vi "MainV1.vi"() -> ()   [LabVIEW 2016]
uses:
  Control/GUICluster.ctl
  Control/Fahrart.ctl
  <vilib>/myRIO/Instrument Drivers/Onboard IO/AI/typedefs/AI Reference.ctl
  <vilib>/myRIO/Common/Instrument Driver Framework/Utilities/typedefs/myRIO Generic Hardware Reference.ctl
  <vilib>/myRIO/Common/Instrument Driver Framework/Utilities/typedefs/Hardware Version Enum.ctl
  <vilib>/myRIO/Common/Instrument Driver Framework/Utilities/typedefs/myRIO v1.0 Reference.ctl
  <vilib>/myRIO/Common/Instrument Driver Framework/Utilities/typedefs/Generic FPGA Reference.ctl
  <vilib>/myRIO/Common/Instrument Driver Framework/myRIO v1.0/AI/typedefs/AI Channels List.ctl
  <vilib>/myRIO/Common/Instrument Driver Framework/myRIO v1.0/AI/typedefs/AI Channels Enum.ctl
  <vilib>/myRIO/Common/Instrument Driver Framework/Utilities/typedefs/Analog Scaling Constants List.ctl
  <vilib>/myRIO/Common/Instrument Driver Framework/Utilities/typedefs/Analog Scaling Constants.ctl
  <vilib>/userdefined/High Color/nirio_resource_hc.ctl
  <vilib>/myRIO/Instrument Drivers/Onboard IO/PWM/typedefs/PWM Reference.ctl
  <vilib>/myRIO/Common/Instrument Driver Framework/myRIO v1.0/PWM/typedefs/PWM Channels Enum.ctl
  <vilib>/myRIO/Instrument Drivers/Onboard IO/PWM/typedefs/PWM Configuration.ctl
  <vilib>/myRIO/Common/Instrument Driver Framework/Utilities/vis/Is FPGA Ref Available.vi
  <vilib>/myRIO/Common/Instrument Driver Framework/myRIO v1.0/AI/vis/myRIO v1.1 Open AI.vi
  <vilib>/myRIO/Instrument Drivers/Onboard IO/AI/vis/Read.vi
  <vilib>/myRIO/Common/Instrument Driver Framework/myRIO v1.0/PWM/vis/myRIO v1.1 Open PWM.vi
  <vilib>/myRIO/Instrument Drivers/Onboard IO/PWM/vis/Set Duty Cycle and Frequency.vi
  <vilib>/myRIO/Common/Instrument Driver Framework/Utilities/vis/Validate Channels.vi
  <vilib>/myRIO/Common/Instrument Driver Framework/myRIO v1.0/AI/vis/myRIO v1.0 Reserve AI.vi
  <vilib>/myRIO/Common/Instrument Driver Framework/myRIO v1.0/PWM/vis/myRIO v1.0 Reserve PWM.vi
  <vilib>/myRIO/Common/Instrument Driver Framework/myRIO v1.0/AI/vis/myRIO v1.0 Build MUX Configuration AI.vi
  <vilib>/myRIO/Common/Instrument Driver Framework/myRIO v1.0/Resource Manager/vis/myRIO v1.0 Reserve Channel List.vi
  <vilib>/myRIO/Common/Instrument Driver Framework/myRIO v1.0/PWM/vis/myRIO v1.0 Build MUX Configuration PWM.vi
  <vilib>/myRIO/Common/Instrument Driver Framework/myRIO v1.0/Resource Manager/vis/myRIO v1.0 Reserve Channel.vi
  <vilib>/myRIO/Common/Instrument Driver Framework/myRIO v1.0/Resource Manager/vis/myRIO v1.0 Unreserve Channel.vi
  <vilib>/myRIO/Common/Instrument Driver Framework/myRIO v1.0/Resource Manager/vis/myRIO v1.0 Create Configuration List.vi
  <vilib>/myRIO/Common/Instrument Driver Framework/myRIO v1.0/Resource Manager/vis/myRIO v1.0 Build Mutex Name.vi
  <vilib>/Utility/VariantDataType/GetNumericInfo.vi
  <vilib>/Utility/error.llb/Error Cluster From Error Code.vi
  <vilib>/myRIO/Common/Instrument Driver Framework/myRIO v1.0/myRIO v1.1 Open.vi
  <vilib>/myRIO/Common/Instrument Driver Framework/Utilities/vis/IO Manager.vi
  <vilib>/myRIO/Common/Instrument Driver Framework/Utilities/vis/Configuration Manager.vi
  <vilib>/myRIO/Common/Instrument Driver Framework/myRIO v1.0/Resource Manager/vis/myRIO v1.0 Configure IO.vi
  <vilib>/myRIO/Common/Instrument Driver Framework/myRIO v1.0/myRIO v1.0 Close.vi
  <vilib>/myRIO/Common/Instrument Driver Framework/myRIO v1.0/PWM/vis/myRIO v1.0 Write PWM.vi
  <vilib>/myRIO/Common/Instrument Driver Framework/myRIO v1.0/AI/vis/myRIO v1.0 Get Scaling Constants AI.vi
  <vilib>/myRIO/Common/Instrument Driver Framework/myRIO v1.0/AI/vis/myRIO v1.0 Read AI.vi
  <vilib>/myRIO/Express VI/Onboard IO/PWM/PWM Express VI.xnode
  <vilib>/myRIO/Instrument Drivers/Onboard IO/PWM/vis/myRIO PWM Open.xnode
  <vilib>/myRIO/Express VI/Onboard IO/AI/AI Express VI.xnode
  <vilib>/myRIO/Instrument Drivers/Onboard IO/AI/vis/myRIO AI Open.xnode
  <vilib>/myRIO/Instrument Drivers/Onboard IO/PWM/PWM.lvlib
  <vilib>/myRIO/Instrument Drivers/Onboard IO/AI/AI.lvlib
panel:
  out "Rundenzeiten":dbl[](array[numeric])
  out "Drehzahl":dbl(knob) scale=0.0..15000.0
  out "Output":dbl[](array[numeric])
  out "Blank Button":bool
  in  "PID gains out 2":T1={"proportional gain (Kc)"=0.71, "integral time (Ti, min)"=2.0, "derivative time (Td, min)"=0.002} {"proportional gain (Kc)" format="%#_10g"; "integral time (Ti, min)" format="%#_10g"; "derivative time (Td, min)" format="%#_10g"}
  out "Impulse pro Minute":dbl
  out "counter":dbl=1170.0
  out "Leistung":dbl=6.577122973792136
  out "Linefollow_Array":bool[](array[boolean])=[FALSE, FALSE, FALSE, FALSE, TRUE, FALSE, FALSE, FALSE]
  # "Minimum"
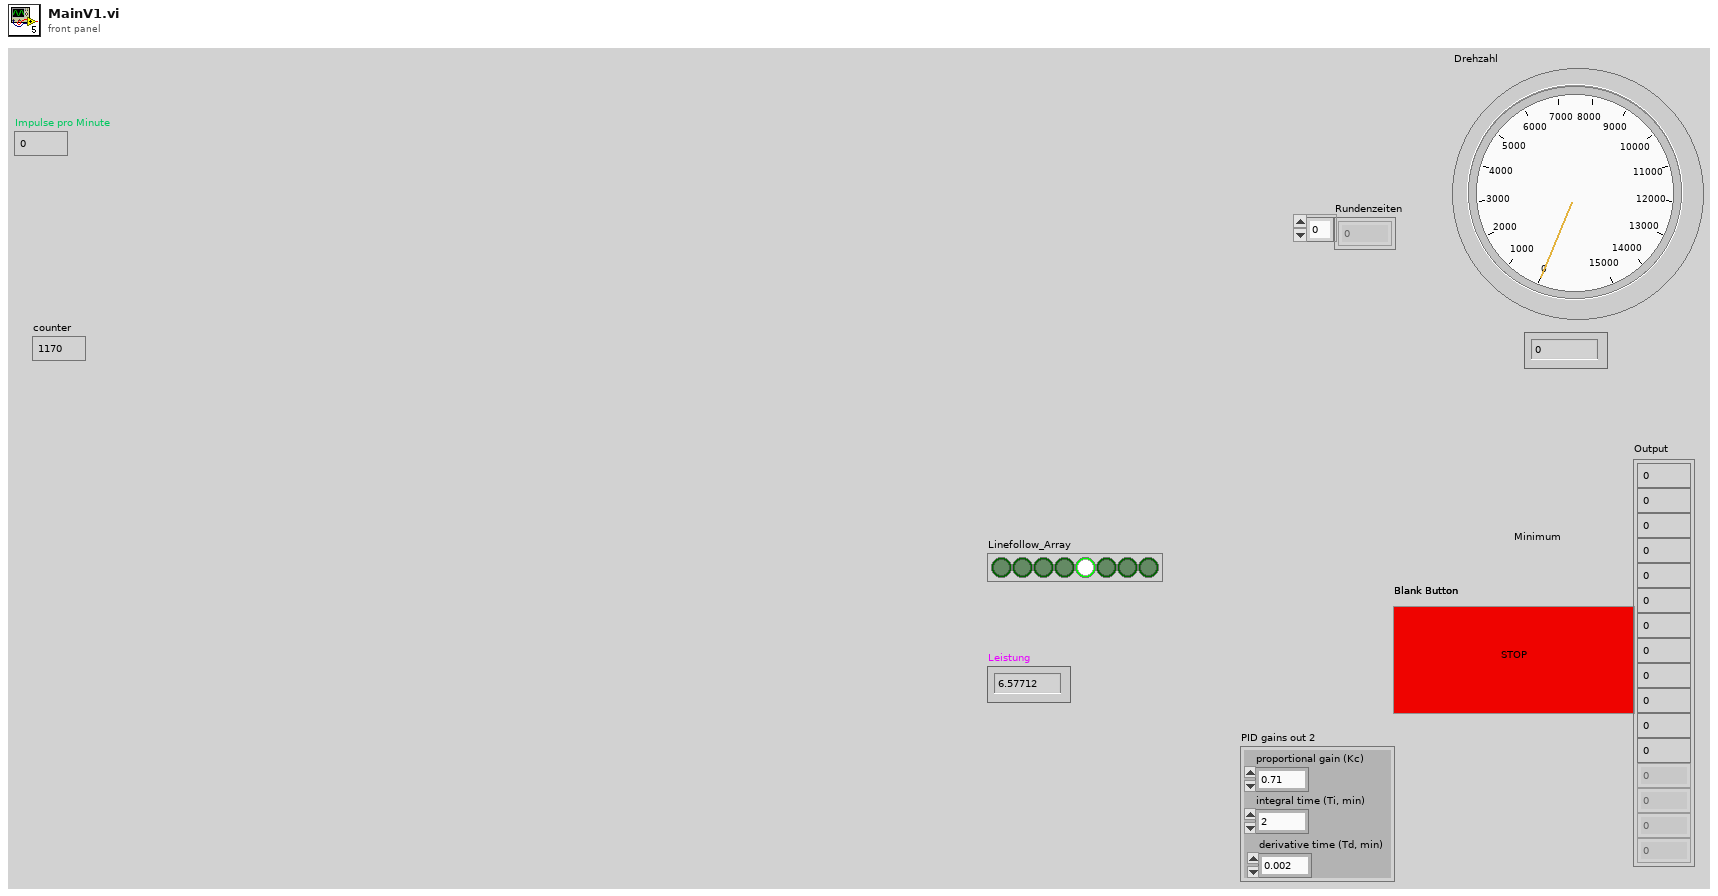
[diagram p1: front panel]
types:
  T1 = cluster{"proportional gain (Kc)":dbl, "integral time (Ti, min)":dbl, "derivative time (Td, min)":dbl}
  T2 = typedef "PWM.lvlib/PWM Reference.ctl" = cluster{"myRIO Reference":T3, "PWM Channels Enum":T7, "PWM Configuration":T8}
  T3 = typedef "myRIO Generic Hardware Reference.ctl" = cluster{"myRIO Model":T4, "myRIO Hardware Reference":T5}
  T4 = typedef "Hardware Version Enum.ctl" = enum16{"Unknown", "myRIO-1900", "myRIO-1950", "roboRIO", "NI ELVIS RIO CM"}
  T5 = typedef "myRIO v1.0 Reference.ctl" = cluster{"Generic FPGA Reference":T6, "Allow multiple opens":bool}
  T6 = typedef "Generic FPGA Reference.ctl" = refnum<k20>
  T7 = typedef "PWM Channels Enum.ctl" = enum16{"Not Connected", "C/PWM0", "C/PWM1", "A/PWM0", "A/PWM1", "A/PWM2", "B/PWM0", "B/PWM1", "B/PWM2", "PWM/PWM0", "PWM/PWM1", "PWM/PWM2", "PWM/PWM3", "PWM/PWM4", "PWM/PWM5", "PWM/PWM6", "PWM/PWM7", "PWM/PWM8", "PWM/PWM9"}
  T8 = typedef "PWM.lvlib/PWM Configuration.ctl" = cluster{"Frequency":dbl, "Duty Cycle":dbl}
  T9 = typedef "nirio_resource_hc.ctl" = tag
  T10 = typedef "GUICluster.ctl" = cluster{"Fahrart":T11, "Geschwindigkeitsmultiplikator":dbl, "Stop":bool}
  T11 = typedef "Fahrart.ctl" = enum16{"Fahren IR", "Fahren Array", "Folgen", "Überholen"}
  T12 = typedef "AI.lvlib/AI Reference.ctl" = cluster{"myRIO Reference":T3, "AI Channels List":T13, "AI Scaling Constants List":T15}
  T13 = typedef "AI Channels List.ctl" = T14[]
  T14 = typedef "AI Channels Enum.ctl" = enum16{"Not Connected", "AudioIn/Left", "AudioIn/Right", "C/AI0", "C/AI1", "A/AI0", "A/AI1", "A/AI2", "A/AI3", "B/AI0", "B/AI1", "B/AI2", "B/AI3", "AI/AI0", "AI/AI1", "AI/AI2", "AI/AI3"}
  T15 = typedef "Analog Scaling Constants List.ctl" = T16[]
  T16 = typedef "Analog Scaling Constants.ctl" = cluster{"LSB Weight (Volts)":dbl, "Offset (Volts)":dbl, "Signed?":bool}
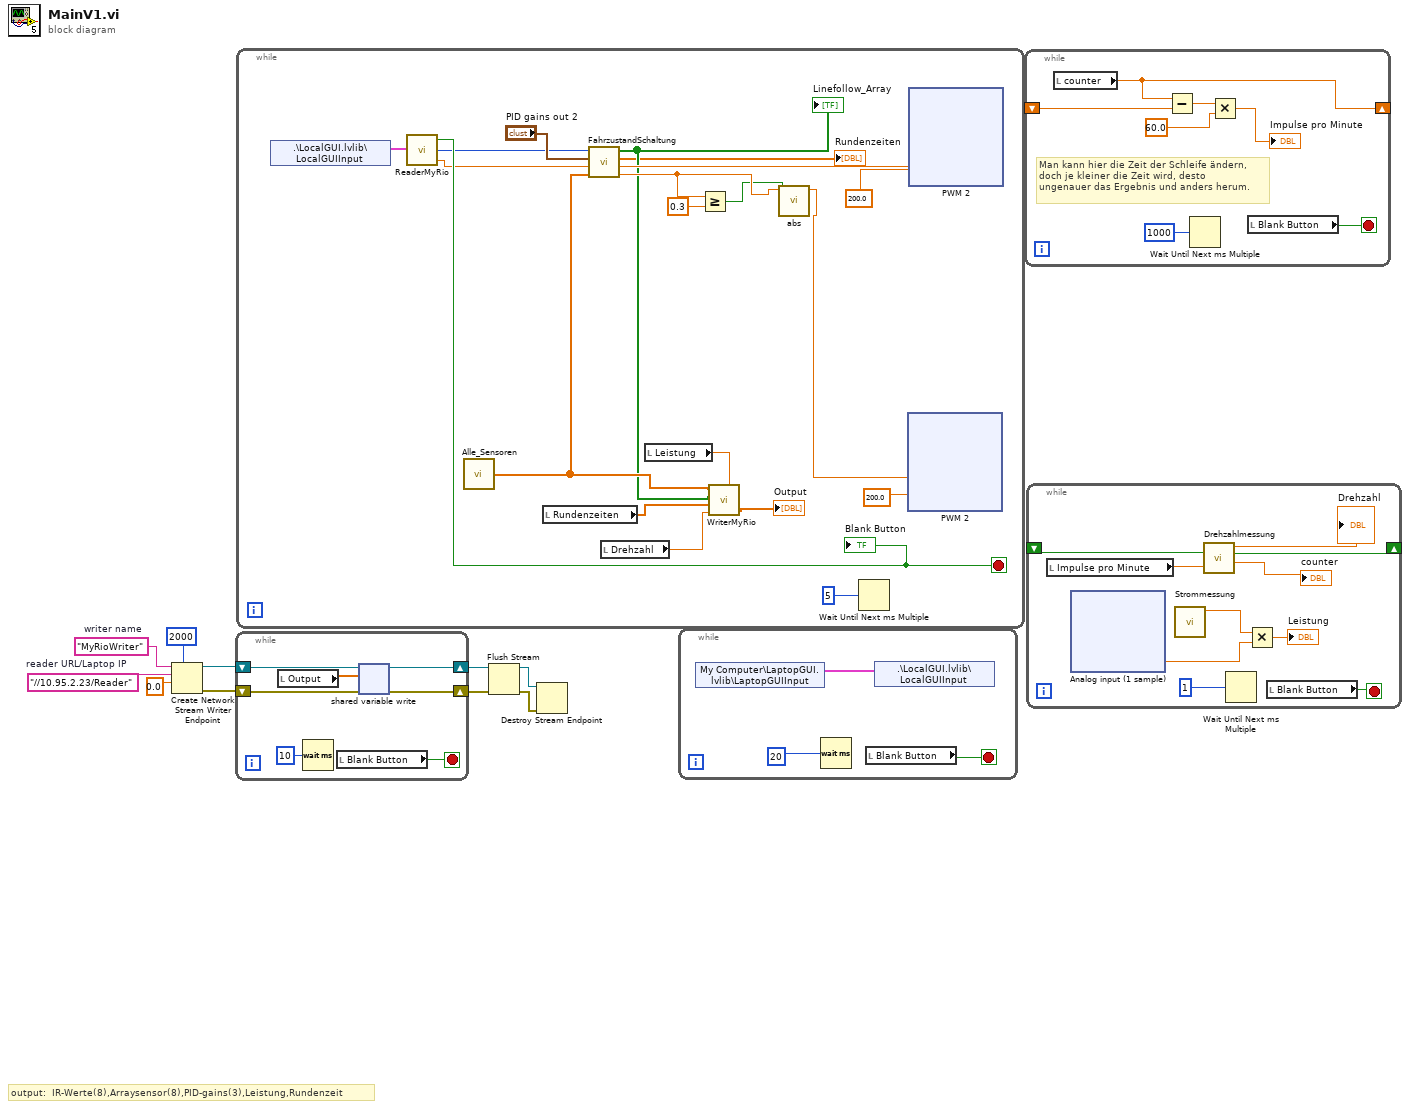
[diagram p0: block diagram]
diagram:
  w9 = "//10.95.2.23/Reader"  # reader URL/Laptop IP
  w10 = "MyRioWriter"  # writer name
  # "output:  IR-Werte(8),Arraysensor(8),PID-gains(3),Leistung,Rundenzeit"
  n1 = Create Network Stream Writer Endpoint(7:2000 ("writer buffer size"), 9:0.0 ("Data Type"), 10:w9, 11:w10) -> (0:w5:errorcluster, 3:w6:refnum<k21>)  [unwired: 3 in]
  n2 = while {
    shift-right: [w14] -> w1
    shift-left: w5 -> [w16]
    shift-right: [w15] -> w2
    shift-left: w6 -> [w17]
    stop <- w11 stop-if-true
    n3 = local read "Output"() -> (w13:dbl[])
    n4 = Wait (ms)(milliseconds to wait=u32 10) -> ()  [unwired: 1 out]
    n5 = local read "Blank Button"() -> (w11:bool)
    n6 = shared-variable-write(w17, w16, w13) -> (w15:refnum<k21>, w14:errorcluster)  [unwired: 1 in, 1 out]
  }
  n7 = while {
    stop <- w33 stop-if-true
    n8 = shared-variable ".\\LocalGUI.lvlib\\LocalGUIInput"() -> (w34:T10)  [unwired: 1 in, 1 out]
    n9 = call "ReaderMyRio.vi"("Cluster"=w34) -> ("Stop"=w33:bool, "Fahrzustand"=w31:T11, "Geschwindigkeitsmultiplikator"=w28:dbl)  [unwired: 1 in]
    "Blank Button" <- w33
    n10 = call "Alle_Sensoren.vi"() -> ("Array"=w24:dbl[])  [unwired: 5 in]
    n11 = local read "Rundenzeiten"() -> (w19:dbl[])
    n12 = call "FahrzustandSchaltung.vi"("Sensoren"=w24, "Geschwindigkeitsmultiplikator"=w28, "PID gains out 2"="PID gains out 2", "Fahrzustand"=w31) -> ("PWM Motor"=w26:dbl, "PWM Lenkung"=w30:dbl, "Rundenzeiten"=→"Rundenzeiten":dbl[], "Linefollow_Array"=w21:bool[])
    "Linefollow_Array" <- w21
    n13 = local read "Drehzahl"() -> (w18:dbl)
    n14 = local read "Leistung"() -> (w23:dbl)
    n15 = Greater Or Equal?(x=w26, y=0.3) -> (x >= y?=w25:bool)
    n16 = call "WriterMyRio.vi"("Leistung"=w23, "Drehzahl"=w18, "Rundenzeit"=w19, "Arraysensor"=w21, "IR Sensoren"=w24) -> ("Output"=→"Output":dbl[])  [unwired: 1 in]
    n17 = call "abs.vi"("Boolean 2"=w25, "PWM_in"=w26) -> ("PWM_out"=w29:dbl)  [unwired: 9 in]
    n18 = Wait Until Next ms Multiple(millisecond multiple=u32 5) -> ()  [unwired: 1 out]
    n19 = xnode "PWM 2"("Duty Cycle"=w29, "Frequency [Hz]"=200.0) -> ()  [unwired: 1 in, 1 out]
    n20 = xnode "PWM 2"("Duty Cycle"=w30, "Frequency [Hz]"=200.0 ("y")) -> ()  [unwired: 1 in, 1 out]
  }
  n21 = Flush Stream(8:w1, 11:w2) -> (0:w4:errorcluster, 3:w3:refnum<k21>)  [unwired: 2 in, 1 out]
  n22 = Destroy Stream Endpoint(8:w4, 11:w3) -> ()  [unwired: 1 out]
  n23 = while {
    stop <- w110 stop-if-true
    n24 = shared-variable "My Computer\\LaptopGUI.lvlib\\LaptopGUIInput"() -> (w109:T10)  [unwired: 1 in, 1 out]
    n25 = Wait (ms)(milliseconds to wait=u32 20) -> ()  [unwired: 1 out]
    n26 = local read "Blank Button"() -> (w110:bool)
    n27 = shared-variable ".\\LocalGUI.lvlib\\LocalGUIInput"(w109) -> ()  [unwired: 1 in, 1 out]
  }
  n28 = while {
    shift-right: [w116] -> _
    shift-left: _ -> [w115]
    stop <- w112 stop-if-true
    # "Man kann hier die Zeit der Schleife ändern, \ndoch je kleiner die Zeit wird, desto\nungenauer das Ergebnis und anders herum."
    n29 = local read "counter"() -> (w116:dbl)
    n30 = Subtract(x=w116, y=w115) -> (x-y=w113:dbl)
    n31 = Wait Until Next ms Multiple(millisecond multiple=u32 1000 ("Vielfache von ms")) -> ()  [unwired: 1 out]
    n32 = Multiply(x=w113, y=60.0) -> (x*y=→"Impulse pro Minute":dbl)
    n33 = local read "Blank Button"() -> (w112:bool)
  }
  n34 = while {
    shift-right: [w120] -> _
    shift-left: _ -> [w119]
    stop <- w121 stop-if-true
    n35 = local read "Impulse pro Minute"() -> (w126:dbl)
    n36 = xnode "Analog input (1 sample)"() -> ("C/AI0 (AI0)"=w124:dbl)  [unwired: 1 in, 1 out]
    n37 = call "Strommessung.vi"() -> ("Strom"=w122:dbl)  [unwired: 10 in, 1 out]
    n38 = call "Drehzahlmessung.vi"("Impuls per Minute"=w126, "in"=w119) -> ("counter"=→"counter":dbl, "out"=w120:bool, "Drehzahl"=→"Drehzahl":dbl)  [unwired: 6 in]
    n39 = Wait Until Next ms Multiple(millisecond multiple=u32 1 ("milliseconds to wait")) -> ()  [unwired: 1 out]
    n40 = Multiply(x=w122, y=w124) -> (x*y=→"Leistung":dbl)
    n41 = local read "Blank Button"() -> (w121:bool)
  }
